vi "Execute State Change Callback.vi"(8 "error in (no error)":errorcluster, 9 "Connection State":bool, 10 "Connection ID":string, 11 "IConnectionStateChangeCallback in":refnum<class "IConnectionStateChangeCallback.lvclass">) -> (0 "error out":errorcluster)   [LabVIEW 2020, in "MessagingInterfaces.lvlib" / "IConnectionStateChangeCallback.lvclass"]
uses:
  <vilib>/gpm_packages/@cs/Network-interface/Source/MessagingInterfaces/IConnectionStateChangeCallback/IConnectionStateChangeCallback.lvclass
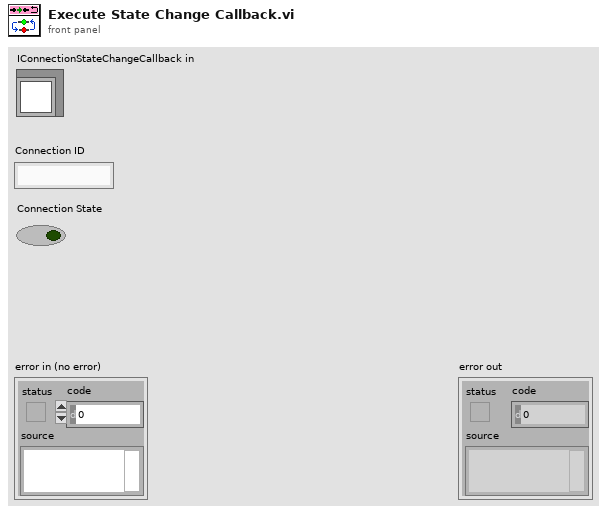
[diagram p1: front panel]
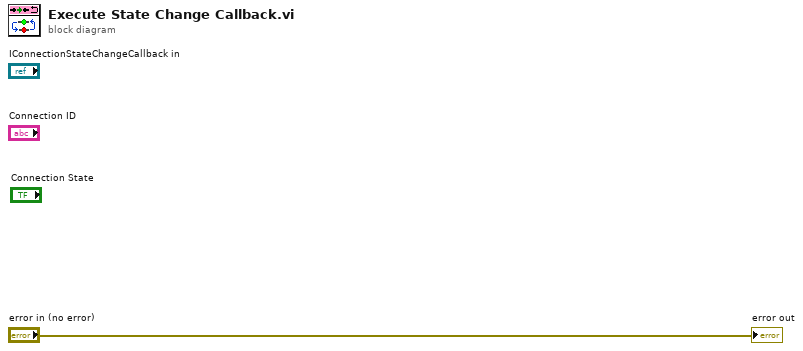
[diagram p0: block diagram]
diagram:
  "error out" <- "error in (no error)"
